vi "读取数据库(子VI).vi"(6 "数据库选择":u16(ring) items=["使用ACCESS数据库", "使用mySQL数据库"], 7 "error in (no error)":errorcluster, 8 "结束日期":string="2020/01/01", 9 "起始日期":string="2010/01/01", 10 "colums":string[](array[string]), 11 "database":string="database1.mdb") -> (0 "错误输出":errorcluster, 1 "表格":string[][](table))   [LabVIEW 2016]
uses:
  <vilib>/Utility/sysdir.llb/System Directory Type.ctl
  <vilib>/addons/database/Connection.llb/DB Tools Open Connec (String).vi
  <vilib>/addons/database/_DB Variant To Data/Database Variant To Data.xnode
  <vilib>/addons/database/NI_Database_API.lvlib
panel:
  out "连接的字符串":string
  out "columns":string[](array[string])
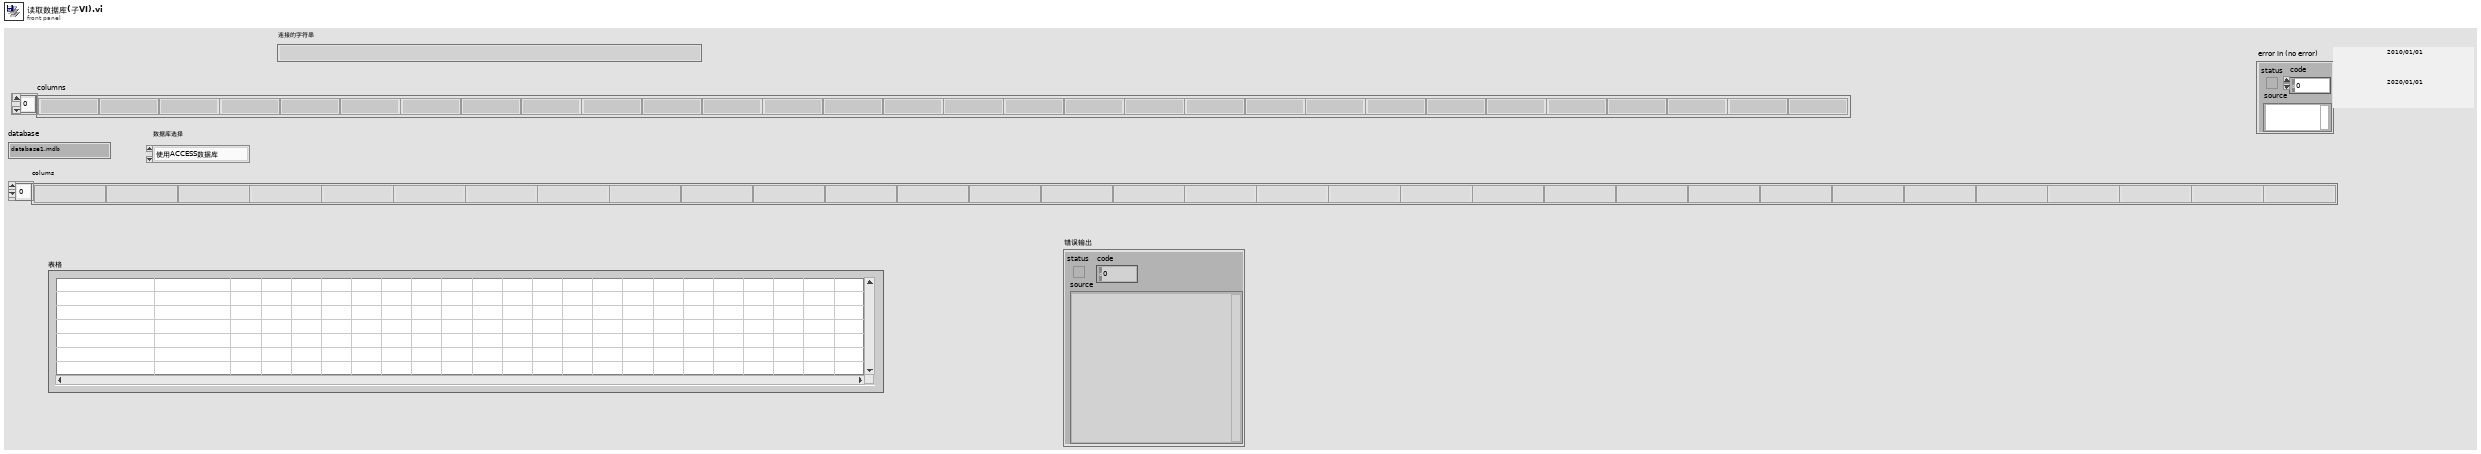
[diagram p1: front panel]
types:
  T1 = typedef "System Directory Type.ctl" = i32
  T2 = typedef "NI_Database_API.lvlib/Conn ObjectReference.ctl" = refnum<k1>
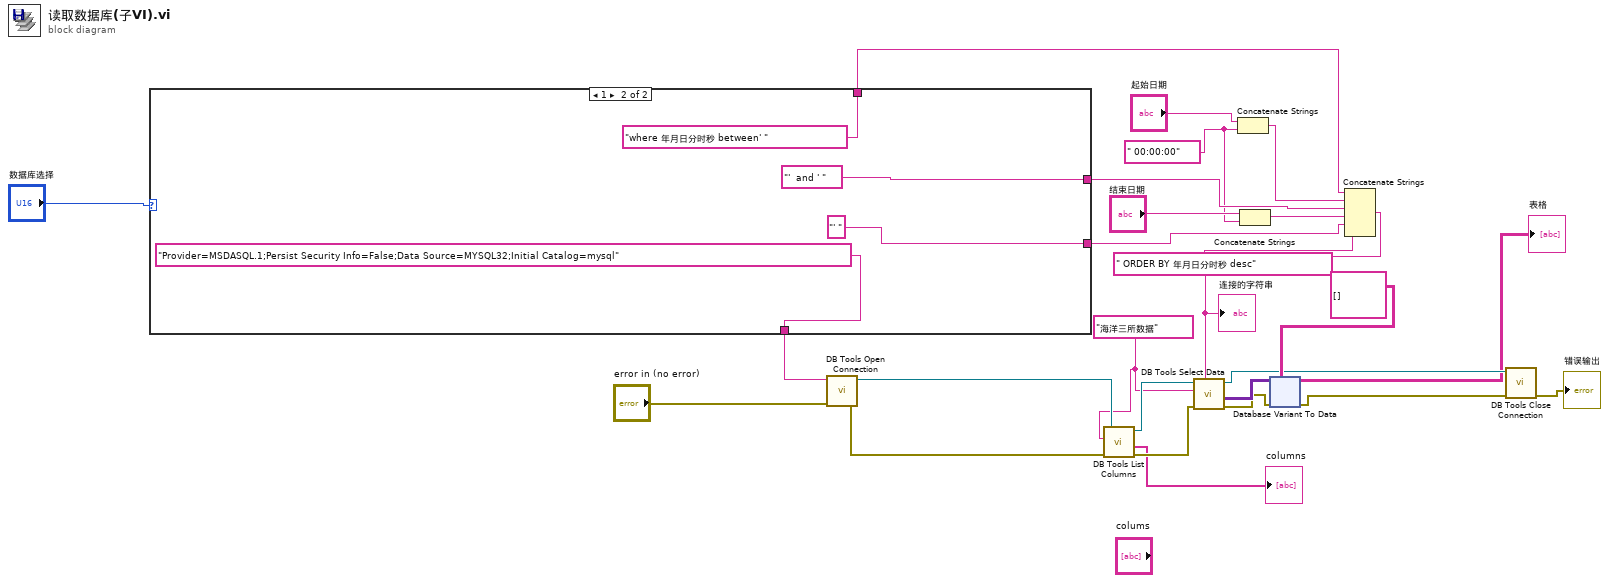
[diagram p0: block diagram]
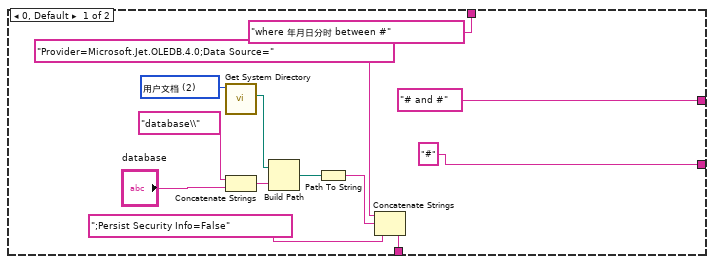
[diagram p2: hidden frame]
diagram:
  w1 = " 00:00:00" ("字符串")
  w13 = "海洋三所数据" ("table")
  n1 = case shown="1" "数据库选择" {
    tunnel: [w39 "Provider=MSDASQL.1;Persist Security Info=False;Data Source=MYSQL32;Initial Catalog=mysql"] -> w25
    tunnel: ["where 年月日分时 between #" "where 年月日分时秒 between' "] -> w8
    tunnel: ["# and #" ("condition") "'  and ' " ("condition")] -> w7
    tunnel: ["#" ("condition") "' " ("condition")] -> w6
    frame 0, Default {
      w31 = T1 2 items=["用户目录"=0, "用户桌面"=1, "用户文档"=2, "用户应用程序数据"=3, "用户设置"=4, "用户临时目录"=5, "公共文档"=6, "公共应用程序数据"=7, "公共设置"=8, "公共缓存"=13, "系统核心库"=9, "系统安装库"=10, "应用程序文件"=11, "启动盘根目录"=12] ("system directory type")
      n2 = call <vilib>:"Get System Directory.vi"("system directory type"=w31) -> ("system directory"=w33:path)  [unwired: 10 in]
      n3 = Concatenate Strings("database\\" ("condition"), "database") -> (w37:string)
      n4 = Build Path(base path=w33, name or relative path=w37) -> (appended path=w34:path)
      n5 = Path To String(path=w34) -> (string=w35:string)
      n6 = Concatenate Strings("Provider=Microsoft.Jet.OLEDB.4.0;Data Source=" ("condition"), w35, ";Persist Security Info=False" ("condition")) -> (w39:string)
    }
    frame 1 {
    }
  }
  n7 = call-poly <vilib>:"DB Tools Open Connection.vi"("error in (no error)"="error in (no error)", "connection information"=w25) -> ("error out"=w12:errorcluster, "connection reference"=w15:T2)  [unwired: 6 in]
  n8 = call <vilib>:"DB Tools List Columns.vi"("error in (no error)"=w12, "table"=w13, "connection reference"=w15) -> ("error out"=w11:errorcluster, "columns"=→"columns":string[], "connection reference out"=w14:T2)  [unwired: 1 in, 1 out]
  n9 = Concatenate Strings("起始日期", w1) -> (w2:string)
  n10 = Concatenate Strings("结束日期", w1) -> (w4:string)
  n11 = Concatenate Strings(w8, w2, w7, w4, w6, " ORDER BY 年月日分时秒 desc" ("字符串")) -> (w16:string)
  "连接的字符串" <- w16
  n12 = call <vilib>:"DB Tools Select Data.vi"("condition"=w16, "error in (no error)"=w11, "table"=w13, "connection reference"=w14) -> ("error out"=w21:errorcluster, "data"=w24:variant[][], "connection reference out"=w19:T2)  [unwired: 2 in]
  n13 = xnode "Database Variant To Data"("database variant"=w24, "error in (no error)"=w21, "type"=string[][] [] ("表格")) -> ("data"=→"表格":string[][], "error out"=w18:errorcluster)
  n14 = call <vilib>:"DB Tools Close Connection.vi"("error in (no error)"=w18, "connection reference"=w19) -> ("error out"=→"错误输出":errorcluster)  [unwired: 5 in]
